vi "Config Check Valid Case Name.vi"(4 "Start With Default":bool, 6 "Get(f) Set(t)":bool, 7 "Ver":u64, 8 "Error":errorcluster, 9 "Case Name":string, 11 "Steer Refs":T1) -> (0 "Error Out":errorcluster, 3 "Steer Refs Out":T1, 5 "Ver Out":u64)   [LabVIEW 2023, in "2024 AdvSwerve_ACT.lvlib"]
uses:
  2024 AdvSwerve_ACT.lvlib
  <vilib>/Rock Robotics/WPI/MotorControl/WPI_MotorControlDeviceRef.ctl
  <vilib>/Rock Robotics/WPI/MotorControl/WPI_MotorControlType.ctl
  <vilib>/Rock Robotics/SystemInterfaces/DIO/FPGA_DIOPWMChannel.ctl
  <vilib>/Rock Robotics/WPI/PWM/WPI_PWMDeadband.ctl
  <vilib>/Rock Robotics/SystemInterfaces/DIO/FPGA_DIOChannel.ctl
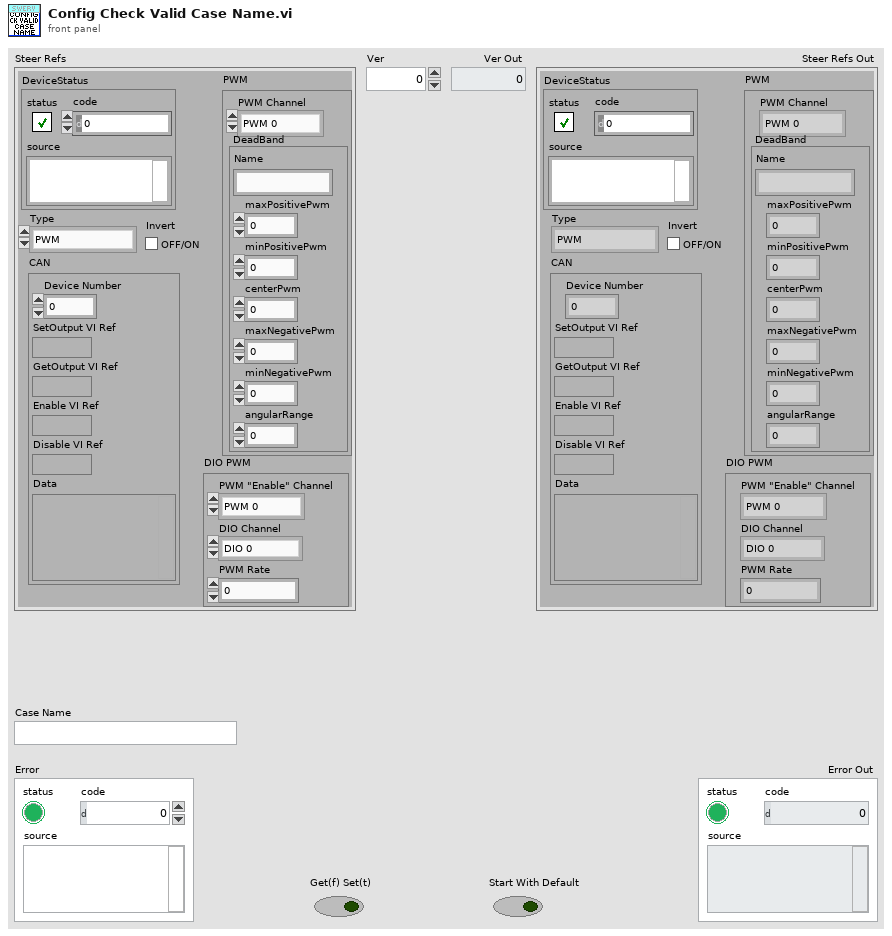
[diagram p1: front panel]
types:
  T1 = typedef "WPI_MotorControlDeviceRef.ctl" = cluster{"DeviceStatus":errorcluster, "Type":T2, "PWM":cluster{"PWM Channel":T3, "DeadBand":T4}, "CAN":cluster{"Device Number":u8, "SetOutput VI Ref":variant, "GetOutput VI Ref":variant, "Enable VI Ref":variant, "Disable VI Ref":variant, "Data":variant}, "Invert":bool, "DIO PWM":cluster{"PWM \"Enable\" Channel":T3, "DIOChannel":T5, "PWM Rate":dbl}}
  T2 = typedef "WPI_MotorControlType.ctl" = enum16{"PWM", "CAN", "DIO PWM"}
  T3 = typedef "FPGA_DIOPWMChannel.ctl" = enum8{"PWM 0", "PWM 1", "PWM 2", "PWM 3", "PWM 4", "PWM 5", "PWM 6", "PWM 7", "PWM 8", "PWM 9", "PWM MXP 0", "PWM MXP 1", "PWM MXP 2", "PWM MXP 3", "PWM MXP 4", "PWM MXP 5", "PWM MXP 6", "PWM MXP 7", "PWM MXP 8", "PWM MXP 9", "Invalid"}
  T4 = typedef "WPI_PWMDeadband.ctl" = cluster{"Name":string, "maxPositivePwm":i32, "minPositivePwm":i32, "centerPwm":i32, "maxNegativePwm":i32, "minNegativePwm":i32, "angularRange":u16}
  T5 = typedef "FPGA_DIOChannel.ctl" = enum8{"DIO 0", "DIO 1", "DIO 2", "DIO 3", "DIO 4", "DIO 5", "DIO 6", "DIO 7", "DIO 8", "DIO 9", "DIO MXP 0", "DIO MXP 1", "DIO MXP 2", "DIO MXP 3", "DIO MXP 4", "DIO MXP 5", "DIO MXP 6", "DIO MXP 7", "DIO MXP 8", "DIO MXP 9", "DIO MXP 10", "DIO MXP 11", "DIO MXP 12", "DIO MXP 13", "DIO MXP 14", "DIO MXP 15", "SPI Port CS1", "SPI Port CS2", "SPI Port CS3", "SPI Port MISO", "SPI Port MOSI", "Invalid"}
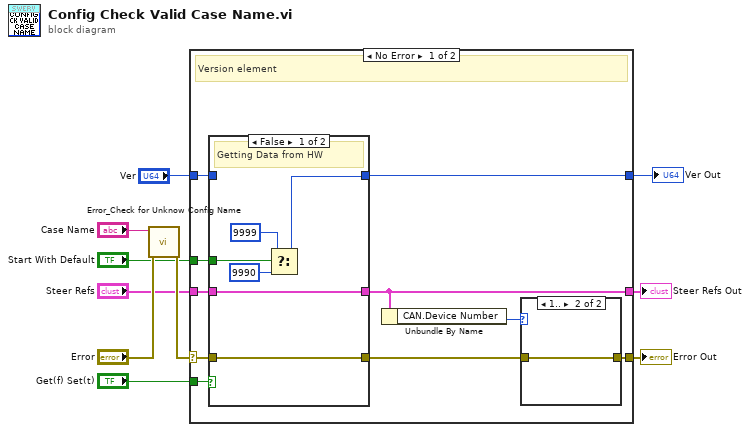
[diagram p0: block diagram]
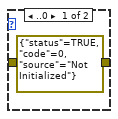
[diagram p2: hidden frame]
diagram:
  n1 = call "Error_Check for Unknow Config Name.vi"("error in (no error)"="Error", "Config Name"="Case Name") -> ("error out"=w7:errorcluster)  [unwired: 9 in]
  n2 = case shown="No Error" w7 {
    selector: w7 -> [w17 w32]
    tunnel: "Steer Refs" -> [w20 w33]
    tunnel: [w14 w33] -> w2
    tunnel: [w12 w32] -> w3
    tunnel: "Get(f) Set(t)" -> [w19 _]
    tunnel: "Start With Default" -> [w18 _]
    tunnel: "Ver" -> [w16 w34]
    tunnel: [w15 w34] -> w10
    frame No Error {
      # "Version element"
      n3 = case shown="False" w19 {
        tunnel: w17 -> [w27 w30]
        tunnel: [w27 w30] -> w11
        tunnel: w20 -> [w28 w31]
        tunnel: [w28 w31] -> w14
        tunnel: w18 -> [w26 _]
        tunnel: w16 -> [_ w29]
        tunnel: [w23 w29] -> w15
        frame False {
          # "Getting Data from HW"
          n4 = Select(t=u64 9999 ("Drive Module Ver"), s=w26, f=u64 9990 ("Drive Module Ver")) -> (s? t:f=w23:u64)
        }
        frame True {
          # "Setting Data To HW"
        }
      }
      n5 = Unbundle By Name(w14) -> ("CAN.Device Number"=w13:u8)
      n6 = case shown="1.." w13 {
        tunnel: [errorcluster {"status"=TRUE, "code"=0, "source"="Not Initialized"} ("error out") w22] -> w12
        tunnel: w11 -> [_ w22]
        frame ..0 {
        }
        frame 1.. {
        }
      }
    }
    frame Error {
      # "Not the Version element and not in case list"
    }
  }
  "Ver Out" <- w10
  "Error Out" <- w3
  "Steer Refs Out" <- w2
